vi "Drive Correction.vi"(1 "Tolerance":dbl=1.0 format="%#_13g", 2 "Min. Power":dbl=0.1 format="%#_13g", 3 "Angle":dbl, 4 "Reset?":bool) -> (0 "Motor Powers":cluster{"RMotor":dbl, "LMotor":dbl})   [LabVIEW 2013]
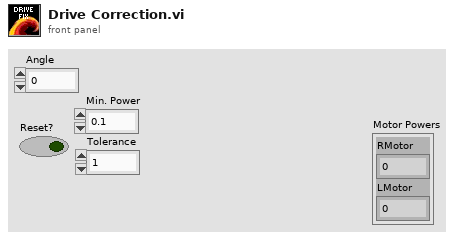
[diagram p1: front panel]
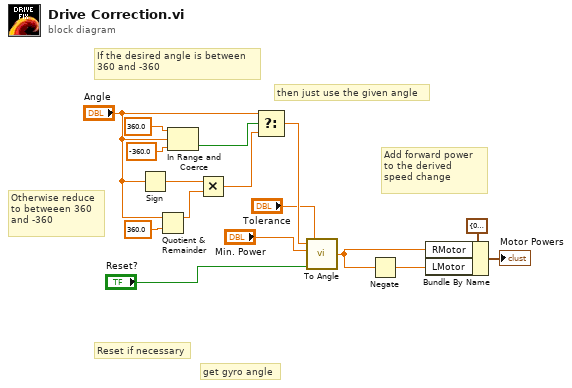
[diagram p0: block diagram]
diagram:
  # "Add forward power\nto the derived\nspeed change"
  # "Reset if necessary"
  # "get gyro angle"
  # "Otherwise reduce\nto betweeen 360\nand -360"
  # "then just use the given angle"
  # "If the desired angle is between \n360 and -360"
  n1 = Sign(1:"Angle") -> (0:w12:dbl)
  n2 = Quotient & Remainder(x="Angle", y=360.0) -> (x-y*floor(x/y)=w13:dbl)  [unwired: 1 out]
  n3 = In Range and Coerce(upper limit=360.0, x="Angle", lower limit=-360.0) -> (In Range?=w8:bool)  [unwired: 1 out]
  n4 = Multiply(x=w12, y=w13) -> (x*y=w6:dbl)
  n5 = Select(t="Angle", s=w8, f=w6) -> (s? t:f=w5:dbl)
  n6 = call "To Angle.vi"("Reset"="Reset?", "Tolerance"="Tolerance", "Min. Power"="Min. Power", "Destination Angle"=w5) -> ("Power Change"=w4:dbl)
  n7 = Negate(x=w4) -> (-x=w3:dbl)
  n8 = Bundle By Name(cluster=cluster{"RMotor":dbl, "LMotor":dbl} {"RMotor"=0.0, "LMotor"=0.0} ("Motor Powers 2"), "RMotor"=w4, "LMotor"=w3) -> (→"Motor Powers":cluster{"RMotor":dbl, "LMotor":dbl})
